vi "FRIC_navX_Internal_SPI_ProcessingLoop.vi"(9 "Clock Rate (Hz)":dbl=2000000.0 format="%_6f", 10 "SPI Bus":T1=enum."Invalid", 11 "Update Rate (4Hz-100Hz)":u8=50 min=4 max=100) -> (0 "error out":errorcluster)   [LabVIEW 2015]
doc: "This navX VI handles the reading/writing for the navX. All of the good stuff is in here.\nTHIS VI SHOULD NOT BE CALLED BY THE USER!"
uses:
  navX Library v2/_TypeDefs/Z900_navX_DeviceTypeDef.ctl
  navX Library v2/_TypeDefs/Z900_navX_ProtocolTypeDef.ctl
  navX Library v2/_TypeDefs/Z900_navX_NotifyPacketTypeDef.ctl
  navX Library v2/_TypeDefs/Z900_navX_ActionTypeDef.ctl
  <vilib>/Rock Robotics/SystemInterfaces/spilib/spi_bus.ctl
  TypeDefs/FRIC_navX_ProcessingLoopStatesTypeDef_I2C.ctl
  TypeDefs/FRIC_navX_I2C Process Loop TypeDef.ctl
  <vilib>/Rock Robotics/SystemInterfaces/Typedef/FPGA_TypedefDigitalModule.ctl
  <vilib>/Rock Robotics/SystemInterfaces/i2clib/i2c_bus.ctl
  navX Library v2/_TypeDefs/Z900_navX_IntegrationControlRegisters.ctl
  <vilib>/Rock Robotics/WPI/SPI/WPI_SPIDevRef.ctl
  _NI WPI Serial USB/WPI_SerialPort_USB.ctl
  navX Library v2/_TypeDefs/Z900_navX_SerialStreamTypeDef.ctl
  <vilib>/Rock Robotics/WPI/SerialPort/WPI_SerialPortRef.ctl
  navX Library v2/_TypeDefs/Flags/Z900_navX_Flags_CapabilityTypeDef.ctl
  navX Library v2/_TypeDefs/Z900_navX_DeviceRegisters.ctl
  navX Library v2/_TypeDefs/navX Open TypeDefs/Z900_navX_OpenTypeDef_SPI.ctl
  <vilib>/Rock Robotics/SystemInterfaces/Utilities/FPGA_UtilitiesRead LocalTime.vi
  navX Library v2/navX Library v2.lvlib
  _NI WPI Serial USB/_NI WPI Serial USB.lvlib
panel:
  out "output cluster":T2={"Interface"={"Protocol"=enum."SERIAL", "Update Rate (4Hz-100Hz)"=4, "navX Open TypeDef"=variant}, "Notify Packet"=refnum, "Loop VI Refnum"=refnum, "Ready to Close Occurrence Refnum"=refnum, "Name"=""} {"Interface"."Update Rate (4Hz-100Hz)" min=4 max=60 step=1}
  out "Connected":bool
  in  "Halt":bool
  out "Registry":u8[](array[numeric])
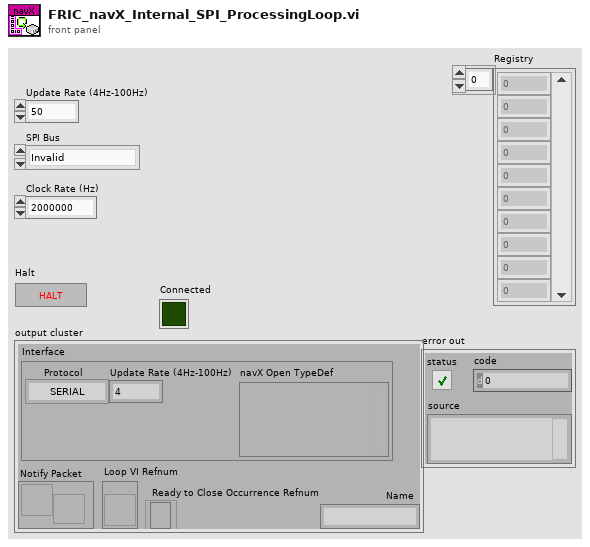
[diagram p1: front panel]
types:
  T1 = typedef "spi_bus.ctl" = enum16{"SPI On-Board, CS0", "SPI On-Board, CS1", "SPI On-Board, CS2", "SPI On-Board, CS3", "SPI MXP", "Invalid"}
  T2 = typedef "navX Library v2.lvlib/Z900_navX_DeviceTypeDef.ctl" = cluster{"Interface":cluster{"Protocol":T3, "Update Rate (4Hz-100Hz)":u8, "navX Open TypeDef":variant}, "Notify Packet":refnum<notifier>, "Loop VI Refnum":refnum<vi>, "Ready to Close Occurrence Refnum":refnum<k4>, "Name":string}
  T3 = typedef "navX Library v2.lvlib/Z900_navX_ProtocolTypeDef.ctl" = enum16{"SERIAL", "I2C", "SPI"}
  T4 = typedef "FRIC_navX_ProcessingLoopStatesTypeDef_I2C.ctl" = enum16{"Process", "INI", "Check Packets Valid", "Close", "Decode Serial Packet", "Flush Serial", "Generate Command", "Last Packet Valid", "Open", "Read", "Reset Serial", "Set Termination Char", "Wait", "Write", "Exit"}
  T5 = typedef "FRIC_navX_I2C Process Loop TypeDef.ctl" = cluster{"State Array":T4[], "error":errorcluster, "FPGA Cluster":cluster{"Last Valid FPGA Time":dbl, "Error Count":i32, "Initialized":bool}, "Device Info":T2, "I2CDevRef":cluster{"DevStatus":errorcluster, "Controller":T6, "Device Address":u8, "Handle":i32, "I2C Bus":T7}, "Registry":u8[], "Command Array":T8[], "Connected?":bool, "navX Device Memory Size":i32, "notification":T9, "Memory Size Set":bool, "SPIDevRef":T11, "navX Serial Open":cluster{"Serial Port":T12, "Stream Type":T13}, "SerialPortRef":T14, "Serial Read Buffer":string, "Serial Write Buffer":string[]}
  T6 = typedef "FPGA_TypedefDigitalModule.ctl" = enum16{"Controller 1"}
  T7 = typedef "i2c_bus.ctl" = enum16{"I2C On-Board", "I2C MXP", "Invalid"}
  T8 = typedef "navX Library v2.lvlib/Z900_navX_IntegrationControlRegisters.ctl" = u8
  T9 = typedef "navX Library v2.lvlib/Z900_navX_NotifyPacketTypeDef.ctl" = cluster{"navX Action":T10, "Data":variant}
  T10 = typedef "navX Library v2.lvlib/Z900_navX_ActionTypeDef.ctl" = enum16{"None", "Halt", "Normal Read", "Update Serial Protocol", "Update Rate Htz", "Zero-Yaw", "Zero-Displacement", "Zero-Velocity"}
  T11 = typedef "WPI_SPIDevRef.ctl" = cluster{"DevStatus":errorcluster, "Handle":i32, "Controller":T6, "SPI Bus":T1}
  T12 = typedef "_NI WPI Serial USB.lvlib/WPI_SerialPort_USB.ctl" = enum16{"Onboard RS-232", "MXP TTL", "USB"}
  T13 = typedef "navX Library v2.lvlib/Z900_navX_SerialStreamTypeDef.ctl" = enum16{"YRPH", "Quaterinons", "Gyro/Raw", "AHRS", "AHRSAndPositioning"}
  T14 = typedef "WPI_SerialPortRef.ctl" = cluster{"DevStatus":errorcluster, "Serial Port Name":refnum<visa-resource-name>}
  T15 = typedef "navX Library v2.lvlib/Z900_navX_OpenTypeDef_SPI.ctl" = cluster{"SPI Bus":T1, "Clock Rate (Hz)":dbl}
  T16 = typedef "navX Library v2.lvlib/Z900_navX_DeviceRegisters.ctl" = u8
  T17 = typedef "navX Library v2.lvlib/Z900_navX_Flags_CapabilityTypeDef.ctl" = u16
  T18 = cluster{"Last Valid FPGA Time":dbl, "Error Count":i32, "Initialized":bool}
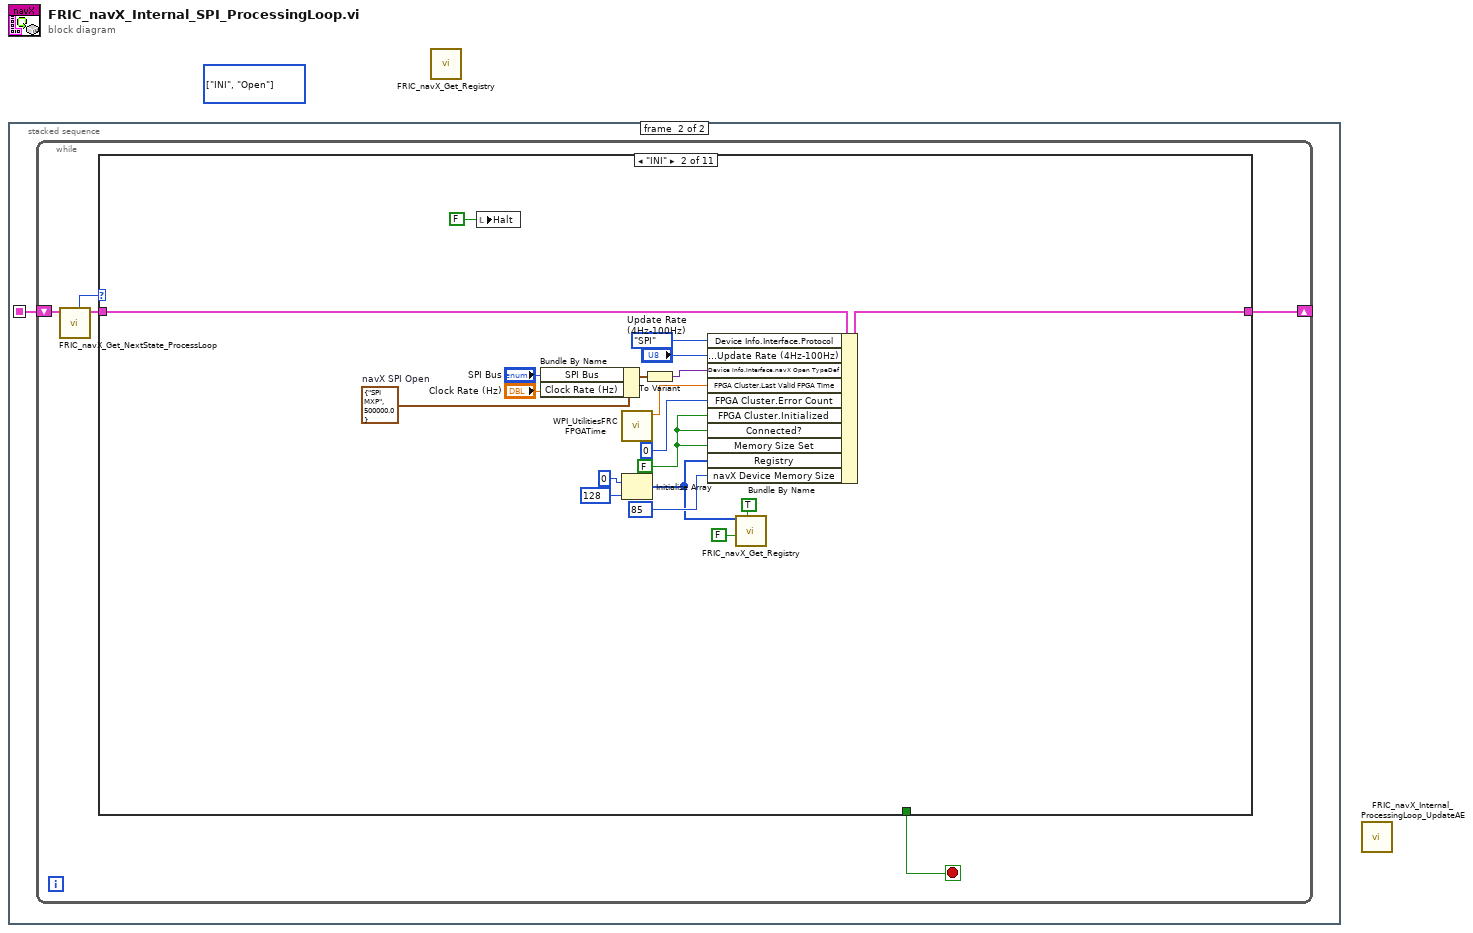
[diagram p0: block diagram]
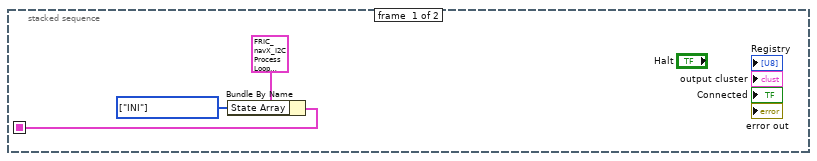
[diagram p2: hidden frame]
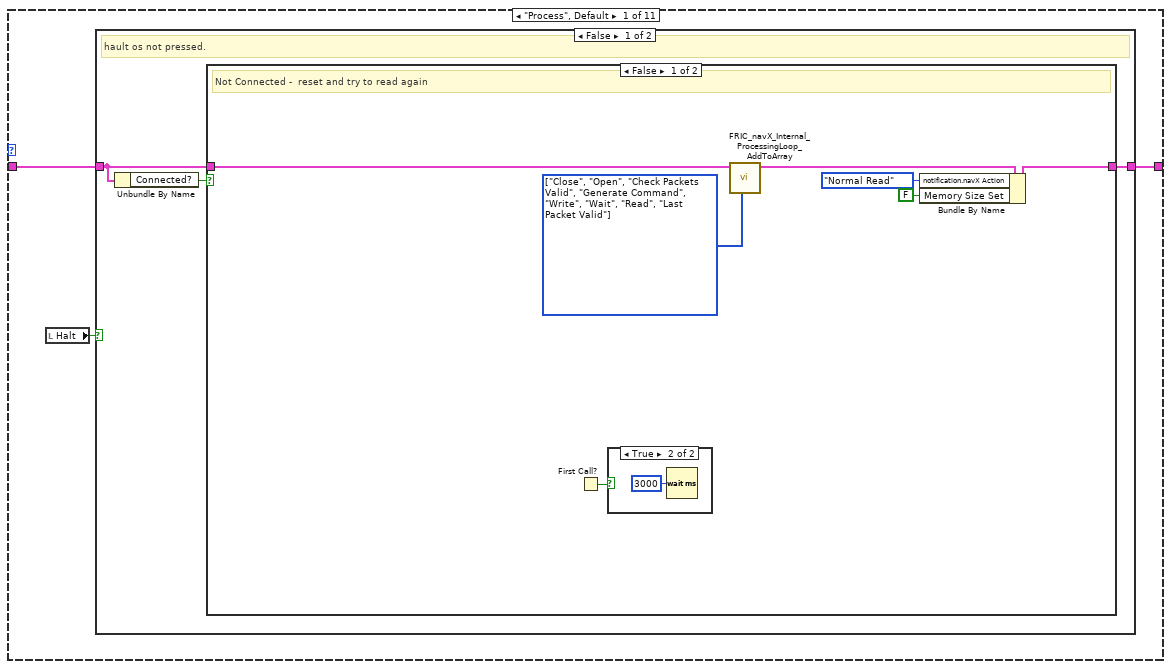
[diagram p3: hidden frame]
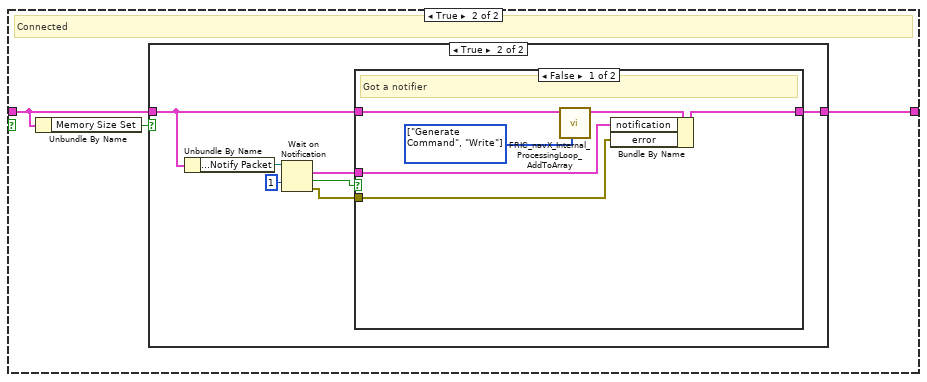
[diagram p5: hidden frame]
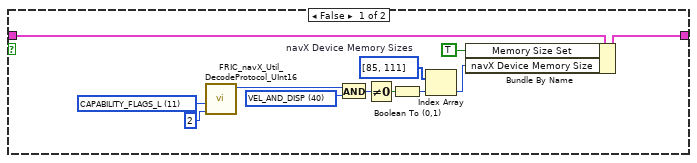
[diagram p6: hidden frame]
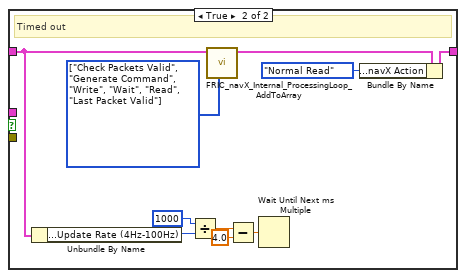
[diagram p7: hidden frame]
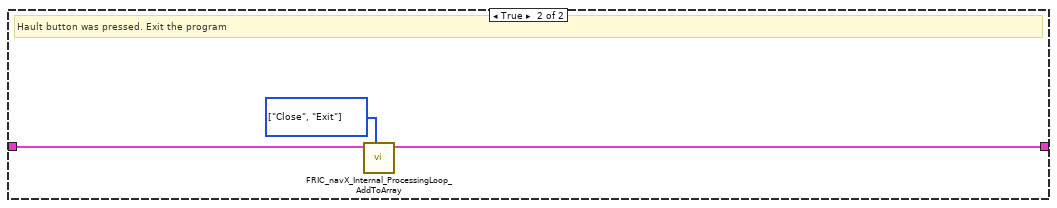
[diagram p8: hidden frame]
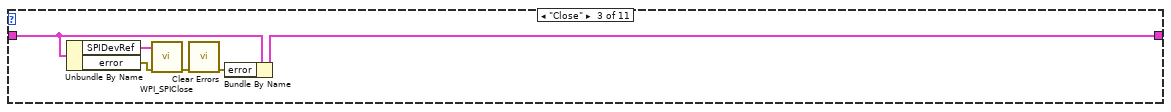
[diagram p9: hidden frame]
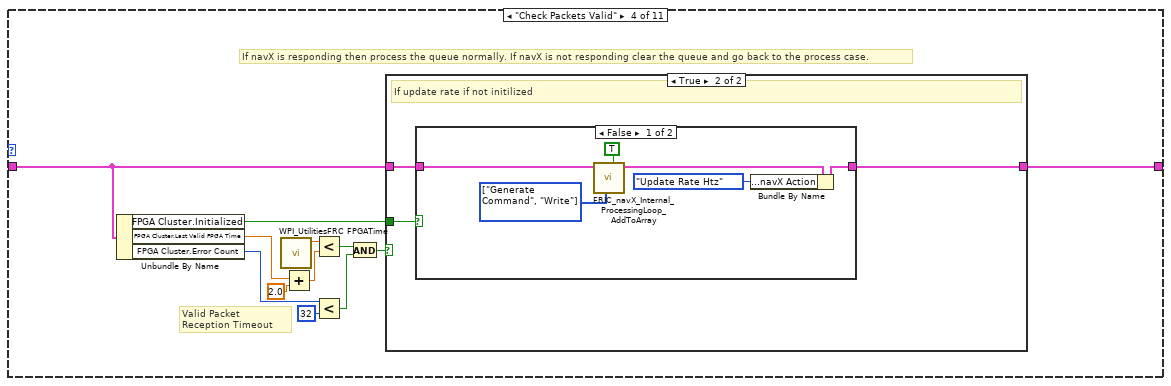
[diagram p10: hidden frame]
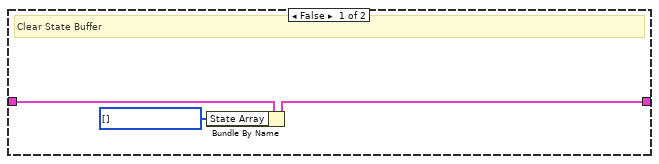
[diagram p11: hidden frame]
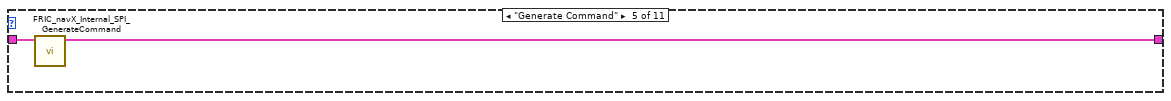
[diagram p13: hidden frame]
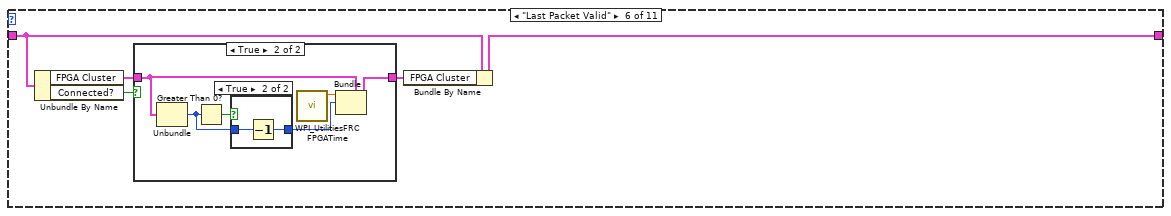
[diagram p14: hidden frame]
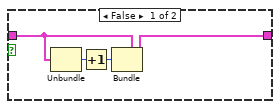
[diagram p15: hidden frame]
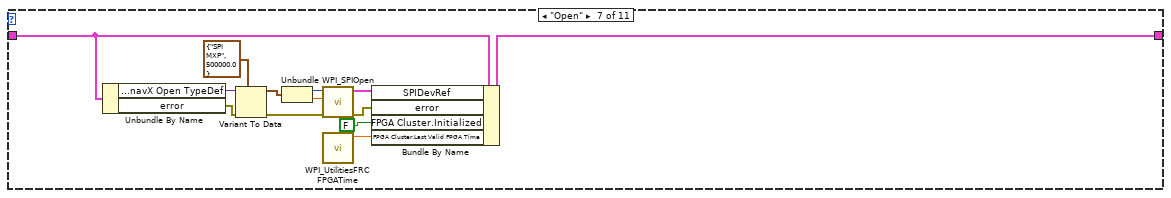
[diagram p17: hidden frame]
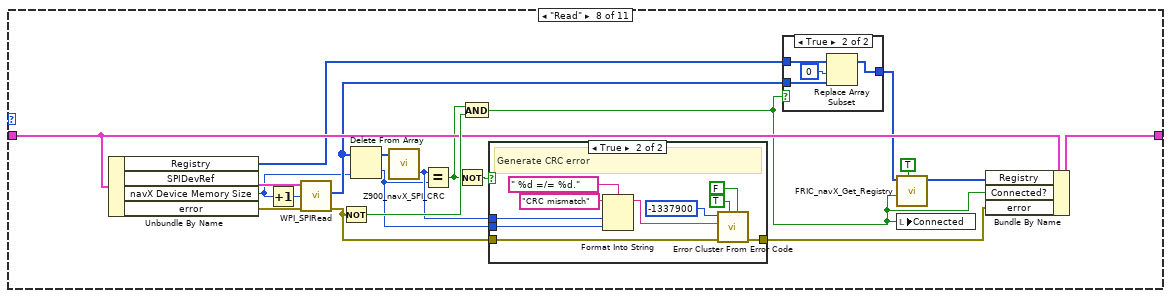
[diagram p18: hidden frame]
diagram:
  (unwired) T4[] [enum."INI", enum."Open"] items=["Process", "INI", "Check Packets Valid", "Close", "Decode Serial Packet", "Flush Serial", "Generate Command", "Last Packet Valid", "Open", "Read", "Reset Serial", "Set Termination Char", "Wait", "Write", "Exit"]
  n1 = stacked-sequence {
    seq-local: [w3 _] -> [_ w4]
    frame #0 {
      w1 = T4[] [enum."INI"] items=["Process", "INI", "Check Packets Valid", "Close", "Decode Serial Packet", "Flush Serial", "Generate Command", "Last Packet Valid", "Open", "Read", "Reset Serial", "Set Termination Char", "Wait", "Write", "Exit"] ("State Array")
      n2 = Bundle By Name(cluster=T5 {"State Array"=[enum."INI", enum."Open"], "error"={"status"=FALSE, "code"=0, "source"=""}, "FPGA Cluster"={"Last Valid FPGA Time"=0.0, "Error Count"=0, "Initialized"=FALSE}, "Device Info"={"Interface"={"Protocol"=enum."SERIAL", "Update Rate (4Hz-100Hz)"=4, "navX Open TypeDef"=variant}, "Notify Packet"=refnum, "Loop VI Refnum"=refnum, "Ready to Close Occurrence Refnum"=refnum, "Name"=""}, "I2CDevRef"={"DevStatus"={"status"=FALSE, "code"=0, "source"=""}, "Controller"=enum."Controller 1", "Device Address"=0, "Handle"=0, "I2C Bus"=enum."Invalid"}, "Registry"=[], "Command Array"=[214, 32], "Connected?"=FALSE, "navX Device Memory Size"=85, "notification"={"navX Action"=enum."None", "Data"=variant}, "Memory Size Set"=FALSE, "SPIDevRef"={"DevStatus"={"status"=FALSE, "code"=0, "source"=""}, "Handle"=0, "Controller"=enum."Controller 1", "SPI Bus"=enum."SPI On-Board, CS0"}, "navX Serial Open"={"Serial Port"=enum."Onboard RS-232", "Stream Type"=enum."YRPH"}, "SerialPortRef"={"DevStatus"={"status"=FALSE, "code"=0, "source"=""}, "Serial Port Name"=""}, "Serial Read Buffer"="", "Serial Write Buffer"=[]} ("I2C Process Loop TypeDef"), "State Array"=w1) -> (w3:T5)
    }
    frame #1 {
      n3 = while {
        shift-right: [w5] -> _
        shift-left: w4 -> [w8]
        stop <- w9 stop-if-true
        n4 = call "FRIC_navX_Get_NextState_ProcessLoop.vi"("I2C Process Loop TypeDef (in)"=w8) -> ("I2C Process Loop TypeDef (out)"=w7:T5, "Current State"=w6:T4)  [unwired: 9 in]
        n5 = case shown="\"INI\"" w6 {
          tunnel: [_ _ _ _ _ _ _ _ _ _ TRUE] -> w9
          tunnel: w7 -> [w11 w79 w89 w93 w116 w120 w145 w165 w185 w191 w194]
          tunnel: [w12 w73 w88 w94 w115 w119 w144 w164 w185 w192 w194] -> w5
          frame "Process", Default {
            n6 = local read "Halt"() -> (w10:bool)
            n7 = case shown="False" w10 {
              tunnel: [w15 w63] -> w12
              tunnel: w11 -> [w13 w64]
              frame False {
                # "hault os not pressed."
                n8 = Unbundle By Name(w13) -> ("Connected?"=w14:bool)
                n9 = case shown="False" w14 {
                  tunnel: w13 -> [w22 w25]
                  tunnel: [w19 w26] -> w15
                  frame False {
                    w21 = T4[] [enum."Close", enum."Open", enum."Check Packets Valid", enum."Generate Command", enum."Write", enum."Wait", enum."Read", enum."Last Packet Valid"] items=["Process", "INI", "Check Packets Valid", "Close", "Decode Serial Packet", "Flush Serial", "Generate Command", "Last Packet Valid", "Open", "Read", "Reset Serial", "Set Termination Char", "Wait", "Write", "Exit"]
                    # "Not Connected -  reset and try to read again"
                    n10 = First Call?() -> (First Call?: T/F=w16:bool)
                    n11 = case shown="True" w16 {
                      frame False {
                      }
                      frame True {
                        n12 = Wait (ms)(milliseconds to wait=u32 3000) -> ()  [unwired: 1 out]
                      }
                    }
                    n13 = call "FRIC_navX_Internal_ProcessingLoop_AddToArray.vi"("States Array"=w21, "I2C Process Loop TypeDef (in)"=w22) -> ("I2C Process Loop TypeDef (out)"=w20:T5)  [unwired: 9 in]
                    n14 = Bundle By Name(cluster=w20, "notification.navX Action"=Z900_navX_ActionTypeDef."Normal Read", "Memory Size Set"=FALSE) -> (w19:T5)
                  }
                  frame True {
                    # "Connected"
                    n15 = Unbundle By Name(w25) -> ("Memory Size Set"=w24:bool)
                    n16 = case shown="True" w24 {
                      tunnel: [w37 w43] -> w26
                      tunnel: w25 -> [w38 w40]
                      frame False {
                        w36 = T16 11 items=["WHOAMI"=0, "HW_REV"=1, "FW_VER_MAJOR"=2, "FW_VER_MINOR"=3, "UPDATE_RATE_HZ"=4, "ACCEL_FSR_G"=5, "GYRO_FSR_DPS"=6, "OP_STATUS"=8, "CAL_STATUS"=9, "SELFTEST_STATUS"=10, "CAPABILITY_FLAGS_L"=11, "CAPABILITY_FLAGS_H"=12, "SENSOR_STATUS"=16, "TIMESTAMP"=18, "YAW"=22, "ROLL"=24, "PITCH"=26, "HEADING"=28, "FUSED_HEADING"=30, "ALTITUDE_I"=32, "ALTITUDE_D"=34, "LINERA_ACC_X"=36, "LINERA_ACC_Y"=38, "LINERA_ACC_Z"=40, "QUAT_W"=42, "QUAT_X"=44, "QUAT_Y"=46, "QUAT_Z"=48, "MPU_TEMP_C"=50, "GYRO_X"=52, "GYRO_Y"=54, "GYRO_Z"=56, "ACC_X"=58, "ACC_Y"=60, "ACC_Z"=62, "MAG_X"=64, "MAG_Y"=66, "MAG_Z"=68, "PRESSURE_I"=70, "PRESSURE_D"=72, "PRESSURE_TEMP"=74, "YAW_OFFSET"=76, "QUAT_OFFSET_W"=78, "QUAT_OFFSET_X"=80, "QUAT_OFFSET_Y"=82, "QUAT_OFFSET_Z"=84, "INTEGRATION_CONTROL"=86, "VELOCITY_X"=88, "VELOCITY_Y"=92, "VELOCITY_Z"=96, "DISPLACMENT_X"=100, "DISPLACMENT_Y"=104, "DISPLACEMENT_Z"=108] ("Device Register")
                        w31 = T17 40 items=["OMNIMOUNT"=4, "OMNIMOUNT_CONFIG_MASK"=38, "VEL_AND_DISP"=40, "YAW_RESET"=80] ("Capability Flag")
                        w32 = i32[] [85, 111]  # navX Device Memory Sizes
                        n17 = call "FRIC_navX_Util_DecodeProtocol_UInt16.vi"("length"=2, "Device Register"=w36) -> ("Value"=w29:u16)  [unwired: 9 in]
                        n18 = And(x=w29, y=w31) -> (x .and. y?=w30:T17)
                        n19 = Not Equal To 0?(x=w30) -> (x != 0?=w33:bool)
                        n20 = Boolean To (0,1)(Boolean=w33) -> (0, 1=w34:i16)
                        n21 = Index Array(array=w32, index=w34) -> (element=w27:i32)
                        n22 = Bundle By Name(cluster=w38, "Memory Size Set"=TRUE, "navX Device Memory Size"=w27) -> (w37:T5)
                      }
                      frame True {
                        n23 = Unbundle By Name(w40) -> ("Device Info.Notify Packet"=w45:refnum<notifier>)
                        n24 = Wait on Notification(notifier=w45, timeout in ms (-1)=1) -> (notification=w42:T9, timed out?=w39:bool, error out=w41:errorcluster)  [unwired: 2 in, 1 out]
                        n25 = case shown="False" w39 {
                          tunnel: w40 -> [w51 w55]
                          tunnel: [w50 w53] -> w43
                          tunnel: w42 -> [w49 _]
                          tunnel: w41 -> [w46 _]
                          frame False {
                            w47 = T4[] [enum."Generate Command", enum."Write"] items=["Process", "INI", "Check Packets Valid", "Close", "Decode Serial Packet", "Flush Serial", "Generate Command", "Last Packet Valid", "Open", "Read", "Reset Serial", "Set Termination Char", "Wait", "Write", "Exit"] ("States Array")
                            # "Got a notifier"
                            n26 = call "FRIC_navX_Internal_ProcessingLoop_AddToArray.vi"("States Array"=w47, "I2C Process Loop TypeDef (in)"=w51) -> ("I2C Process Loop TypeDef (out)"=w48:T5)  [unwired: 9 in]
                            n27 = Bundle By Name(cluster=w48, "notification"=w49, "error"=w46) -> (w50:T5)
                          }
                          frame True {
                            w56 = T4[] [enum."Check Packets Valid", enum."Generate Command", enum."Write", enum."Wait", enum."Read", enum."Last Packet Valid"] items=["Process", "INI", "Check Packets Valid", "Close", "Decode Serial Packet", "Flush Serial", "Generate Command", "Last Packet Valid", "Open", "Read", "Reset Serial", "Set Termination Char", "Wait", "Write", "Exit"]
                            # "Timed out"
                            n28 = Unbundle By Name(w55) -> ("Device Info.Interface.Update Rate (4Hz-100Hz)"=w61:u8)
                            n29 = Divide(x=i16 1000, y=w61) -> (x/y=w59:dbl)
                            n30 = call "FRIC_navX_Internal_ProcessingLoop_AddToArray.vi"("States Array"=w56, "I2C Process Loop TypeDef (in)"=w55) -> ("I2C Process Loop TypeDef (out)"=w54:T5)  [unwired: 9 in]
                            n31 = Subtract(x=w59, y=4.0) -> (x-y=w57:dbl)
                            n32 = Wait Until Next ms Multiple(millisecond multiple=w57) -> ()  [unwired: 1 out]
                            n33 = Bundle By Name(cluster=w54, "notification.navX Action"=Z900_navX_ActionTypeDef."Normal Read") -> (w53:T5)
                          }
                        }
                      }
                    }
                  }
                }
              }
              frame True {
                w62 = T4[] [enum."Close", enum."Exit"] items=["Process", "INI", "Check Packets Valid", "Close", "Decode Serial Packet", "Flush Serial", "Generate Command", "Last Packet Valid", "Open", "Read", "Reset Serial", "Set Termination Char", "Wait", "Write", "Exit"] ("States Array")
                # "Hault button was pressed. Exit the program"
                n34 = call "FRIC_navX_Internal_ProcessingLoop_AddToArray.vi"("States Array"=w62, "I2C Process Loop TypeDef (in)"=w64) -> ("I2C Process Loop TypeDef (out)"=w63:T5)  [unwired: 9 in]
              }
            }
          }
          frame "INI" {
            w70 = T15 {"SPI Bus"=enum."SPI MXP", "Clock Rate (Hz)"=500000.0}  # navX SPI Open
            w71 = FALSE ("Initialized")
            n35 = local write "Halt"(FALSE ("Halt")) -> ()
            n36 = Bundle By Name(cluster=w70, "SPI Bus"="SPI Bus", "Clock Rate (Hz)"="Clock Rate (Hz)") -> (w80:T15)
            n37 = call <vilib>:"WPI_UtilitiesFRC FPGATime.vi"() -> ("FPGA Time"=w75:dbl)  [unwired: 10 in, 1 out]
            n38 = Initialize Array(u8 0 ("Received Data"), 128 ("hex")) -> (w66:u8[])
            n39 = To Variant(anything=w80) -> (Variant=w76:variant)
            n40 = Bundle By Name(cluster=w79, "Device Info.Interface.Protocol"=Z900_navX_ProtocolTypeDef."SPI" ("Protocol"), "Device Info.Interface.Update Rate (4Hz-100Hz)"="Update Rate (4Hz-100Hz)", "Device Info.Interface.navX Open TypeDef"=w76, "FPGA Cluster.Last Valid FPGA Time"=w75, "FPGA Cluster.Error Count"=0 ("Error Count"), "FPGA Cluster.Initialized"=w71, "Connected?"=w71, "Memory Size Set"=w71, "Registry"=w66, "navX Device Memory Size"=85 ("hex")) -> (w73:T5)
            n41 = call "FRIC_navX_Get_Registry.vi"("Update"=TRUE, "Connected?"=FALSE, "Registry (in)"=w66) -> ()  [unwired: 7 in, 2 out]
          }
          frame "Close" {
            n42 = Unbundle By Name(w89) -> ("SPIDevRef"=w87:T11, "error"=w86:errorcluster)
            n43 = call <vilib>:"WPI_SPIClose.vi"("error in (no error)"=w86, "SPIDevRef"=w87) -> ("error out"=w85:errorcluster)  [unwired: 9 in]
            n44 = call <vilib>:"Clear Errors.vi"("error in (no error)"=w85) -> ("error out"=w84:errorcluster)  [unwired: 5 in, 1 out]
            n45 = Bundle By Name(cluster=w89, "error"=w84) -> (w88:T5)
          }
          frame "Check Packets Valid" {
            # "If navX is responding then process the queue normally. If navX is not responding clear the queue and go back to the process case."
            # "Valid Packet Reception Timeout"
            n46 = Unbundle By Name(w93) -> ("FPGA Cluster.Initialized"=w91:bool, "FPGA Cluster.Last Valid FPGA Time"=w92:dbl, "FPGA Cluster.Error Count"=w90:i32)
            n47 = call <vilib>:"WPI_UtilitiesFRC FPGATime.vi"() -> ("FPGA Time"=w99:dbl)  [unwired: 10 in, 1 out]
            n48 = Add(x=w92, y=2.0) -> (x+y=w100:dbl)
            n49 = Less?(x=w99, y=w100) -> (x < y?=w97:bool)
            n50 = Less?(x=w90, y=32) -> (x < y?=w96:bool)
            n51 = And(x=w97, y=w96) -> (x .and. y?=w95:bool)
            n52 = case shown="True" w95 {
              tunnel: w93 -> [w104 w107]
              tunnel: [w103 w106] -> w94
              tunnel: w91 -> [_ w105]
              frame False {
                w102 = T4[] [] items=["Process", "INI", "Check Packets Valid", "Close", "Decode Serial Packet", "Flush Serial", "Generate Command", "Last Packet Valid", "Open", "Read", "Reset Serial", "Set Termination Char", "Wait", "Write", "Exit"] ("f")
                # "Clear State Buffer"
                n53 = Bundle By Name(cluster=w104, "State Array"=w102) -> (w103:T5)
              }
              frame True {
                # "If update rate if not initilized"
                n54 = case shown="False" w105 {
                  tunnel: w107 -> [w112 w114]
                  tunnel: [w110 w114] -> w106
                  frame False {
                    w108 = T4[] [enum."Generate Command", enum."Write"] items=["Process", "INI", "Check Packets Valid", "Close", "Decode Serial Packet", "Flush Serial", "Generate Command", "Last Packet Valid", "Open", "Read", "Reset Serial", "Set Termination Char", "Wait", "Write", "Exit"] ("f")
                    n55 = call "FRIC_navX_Internal_ProcessingLoop_AddToArray.vi"("Add to beginning"=TRUE, "States Array"=w108, "I2C Process Loop TypeDef (in)"=w112) -> ("I2C Process Loop TypeDef (out)"=w111:T5)  [unwired: 8 in]
                    n56 = Bundle By Name(cluster=w111, "notification.navX Action"=Z900_navX_ActionTypeDef."Update Rate Htz") -> (w110:T5)
                  }
                  frame True {
                  }
                }
              }
            }
          }
          frame "Generate Command" {
            n57 = call "FRIC_navX_Internal_SPI_GenerateCommand.vi"("I2C Process Loop TypeDef (in)"=w116) -> ("I2C Process Loop TypeDef (out)"=w115:T5)  [unwired: 10 in]
          }
          frame "Last Packet Valid" {
            n58 = Unbundle By Name(w120) -> ("FPGA Cluster"=w121:T18, "Connected?"=w117:bool)
            n59 = case shown="True" w117 {
              tunnel: [w124 w131] -> w118
              tunnel: w121 -> [w123 w127]
              frame False {
                n60 = Unbundle(w123) -> ("Error Count"=w122:i32)  [unwired: 2 out]
                n61 = Increment(x=w122) -> (x+1=w125:i32)
                n62 = Bundle(cluster=w123, "Error Count"=w125) -> (w124:T18)  [unwired: 2 in]
              }
              frame True {
                n63 = Unbundle(w127) -> ("Error Count"=w126:i32)  [unwired: 2 out]
                n64 = Greater Than 0?(x=w126) -> (x > 0?=w129:bool)
                n65 = case shown="True" w129 {
                  tunnel: [w132 w134] -> w128
                  tunnel: w126 -> [w132 w133]
                  frame False {
                  }
                  frame True {
                    n66 = Decrement(x=w133) -> (x-1=w134:i32)
                  }
                }
                n67 = call <vilib>:"WPI_UtilitiesFRC FPGATime.vi"() -> ("FPGA Time"=w130:dbl)  [unwired: 10 in, 1 out]
                n68 = Bundle(cluster=w127, "Last Valid FPGA Time"=w130, "Error Count"=w128) -> (w131:T18)  [unwired: 1 in]
              }
            }
            n69 = Bundle By Name(cluster=w120, "FPGA Cluster"=w118) -> (w119:T5)
          }
          frame "Open" {
            n70 = Unbundle By Name(w145) -> ("Device Info.Interface.navX Open TypeDef"=w147:variant, "error"=w143:errorcluster)
            n71 = Variant To Data(error in=w143, type=T15 {"SPI Bus"=enum."SPI MXP", "Clock Rate (Hz)"=500000.0} ("navX SPI Open"), Variant=w147) -> (data=w146:T15, error out=w137:errorcluster)
            n72 = Unbundle(w146) -> ("SPI Bus"=w140:T1, "Clock Rate (Hz)"=w139:dbl)
            n73 = call <vilib>:"WPI_SPIOpen.vi"("error in"=w137, "Clock Rate (Hz)"=w139, "SPI Bus"=w140) -> ("error out"=w136:errorcluster, "SPIDevRef"=w138:T11)  [unwired: 7 in]
            n74 = call <vilib>:"WPI_UtilitiesFRC FPGATime.vi"() -> ("FPGA Time"=w135:dbl)  [unwired: 10 in, 1 out]
            n75 = Bundle By Name(cluster=w145, "SPIDevRef"=w138, "error"=w136, "FPGA Cluster.Initialized"=FALSE ("Initialized"), "FPGA Cluster.Last Valid FPGA Time"=w135) -> (w144:T5)
          }
          frame "Read" {
            n76 = Unbundle By Name(w165) -> ("Registry"=w161:u8[], "SPIDevRef"=w160:T11, "navX Device Memory Size"=w149:i32, "error"=w159:errorcluster)
            n77 = Increment(x=w149) -> (x+1=w148:i32)
            n78 = call <vilib>:"WPI_SPIRead.vi"("error in (no error)"=w159, "Num to Read"=w148, "SPIDevRef"=w160) -> ("error out"=w154:errorcluster, "Received Data"=w157:u8[])  [unwired: 6 in, 1 out]
            n79 = Not(x=w154) -> (.not. x?=w166:bool)
            n80 = Delete From Array(array=w157, index=w149) -> (deleted portion=w151:u8, array with subset deleted=w158:u8[])  [unwired: 1 in]
            n81 = call "Z900_navX_SPI_CRC.vi"("Message"=w158) -> ("CRC"=w152:u8)  [unwired: 1 out]
            n82 = Equal?(x=w152, y=w151) -> (x = y?=w155:bool)
            n83 = Not(x=w155) -> (.not. x?=w150:bool)
            n84 = And(x=w155, y=w166) -> (x .and. y?=w162:bool)
            n85 = case shown="True" w150 {
              tunnel: w152 -> [_ w176]
              tunnel: w151 -> [_ w175]
              tunnel: w154 -> [w168 w172]
              tunnel: [w168 w171] -> w153
              frame False {
              }
              frame True {
                # "Generate CRC error"
                n86 = Format Into String(format string=" %d =/= %d.", initial string="CRC mismatch", w176, w175) -> (resulting string=w173:string)  [unwired: 1 in, 1 out]
                n87 = call <vilib>:"Error Cluster From Error Code.vi"("is warning? (False)"=FALSE, "show call chain? (False)"=TRUE, "error in (no error)"=w172, "error message (\"\")"=w173, "error code (0)"=-1337900 ("code")) -> ("error out"=w171:errorcluster)  [unwired: 4 in]
              }
            }
            n88 = case shown="True" w162 {
              tunnel: w161 -> [w179 w183]
              tunnel: [w179 w182] -> w156
              tunnel: w157 -> [_ w181]
              frame False {
              }
              frame True {
                n89 = Replace Array Subset(array=w183, new element=w181, index=u8 0 ("hex")) -> (w182:u8[])
              }
            }
            n90 = call "FRIC_navX_Get_Registry.vi"("Update"=TRUE, "Connected?"=w162, "Registry (in)"=w156) -> ("Registry (out)"=w163:u8[])  [unwired: 7 in, 1 out]
            n91 = local write "Connected"(w162) -> ()
            n92 = Bundle By Name(cluster=w165, "Registry"=w163, "Connected?"=w162, "error"=w153) -> (w164:T5)
          }
          frame "Wait" {
            n93 = Wait (ms)(milliseconds to wait=u32 1) -> ()  [unwired: 1 out]
          }
          frame "Write" {
            n94 = Unbundle By Name(w191) -> ("SPIDevRef"=w190:T11, "Command Array"=w189:T8[], "I2CDevRef.DevStatus"=w188:errorcluster)
            n95 = call <vilib>:"WPI_SPIWrite.vi"("error in (no error)"=w188, "Data To Send"=w189, "SPIDevRef"=w190) -> ("error out"=w187:errorcluster, "SPIDevRef"=w186:T11)  [unwired: 6 in, 1 out]
            n96 = Bundle By Name(cluster=w191, "SPIDevRef"=w186, "error"=w187) -> (w192:T5)
          }
          frame "Exit" {
            n97 = Unbundle By Name(w194) -> ("Device Info"=w193:T2)
            n98 = in-place {
              in-place-border: [TRUE] -> w196
              in-place-border: w193 -> [w197]
              # "Set Occurence of Close"
              n99 = Unbundle By Name(w197) -> ("Ready to Close Occurrence Refnum"=w199:refnum<k4>)
              n100 = local write "Halt"(FALSE ("Halt")) -> ()
              n101 = Set Occurrence(w199) -> ()
            }
            n102 = Stop(stop? (T)=w196) -> ()
          }
        }
      }
    }
  }
  n103 = call "FRIC_navX_Get_Registry.vi"() -> ()  [unwired: 10 in, 2 out]
  n104 = call "FRIC_navX_Internal_ProcessingLoop_UpdateAE.vi"() -> ()  [unwired: 6 in, 10 out]
